vi "Set Offset.vi"(8 "error in (no error)":errorcluster, 11 "NeedleValve in":refnum<class "NeedleValve.lvclass">) -> (0 "error out":errorcluster, 3 "NeedleValve out":refnum<class "NeedleValve.lvclass">)   [LabVIEW 2019, in "NeedleValve.lvclass"]
uses:
  NeedleValve.lvclass
  NeedleValve.lvclass/NeedleValve.ctl
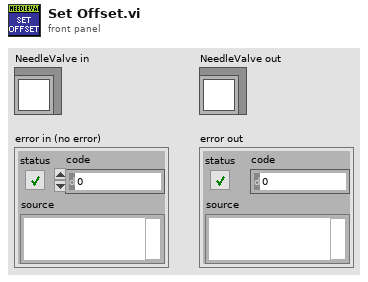
[diagram p1: front panel]
types:
  T1 = typedef "Needle Valve Data.ctl" = cluster{"Engine State":T2, "StateValveModbus":T3, "Alarms":T4, "RAW":i32, "Angele":dbl, "Step":i32, "Encoder":i32, "Kinematic":T5, "Limits":T6, "EncoderMax":i32, "Counter Max Dont Update":i32, "EncoderMin":i32, "Counter Min Dont Update":i32, "Prepere Counter":i32, "STEP INIT":i32, "offset - Angel":dbl}
  T2 = typedef "MB_ENGINE.lvclass/Engine State.ctl" = u16
  T3 = typedef "Needle Valve State.ctl" = enum16{"STOPED", "CLOSED", "OPENED", "OPENING", "CLOSING", "FULL_CLOSE", "PREP_OPEN"}
  T4 = typedef "MB_ENGINE.lvclass/Engine Alarms.ctl" = cluster{"OL":bool, "TF":bool, "STL":bool, "OCP":bool, "CPUV":bool, "UVLO":bool, "SPI_ERROR":bool, "Fault":bool, "OL 2":bool, "TF 2":bool, "STL 2":bool, "OCP 2":bool, "CPUV 2":bool, "UVLO 2":bool, "reserved":bool, "InitDone":bool}
  T5 = typedef "MB_ENGINE.lvclass/Settings.ctl" = cluster{"ACC Steps Per Sec^2":u16, "DEC Steps Per Sec^2":u16, "Min Velosity Step Per Sec":u16, "Max Velosity Step Per Sec":u16, "MicroStep":u16}
  T6 = typedef "MB_ENGINE.lvclass/Limits Status.ctl" = cluster{"Fault 2 Switch":bool, "Fault 1 Switch":bool, "Center(Home)":bool, "Lower Limit":bool, "Upper Limit":bool}
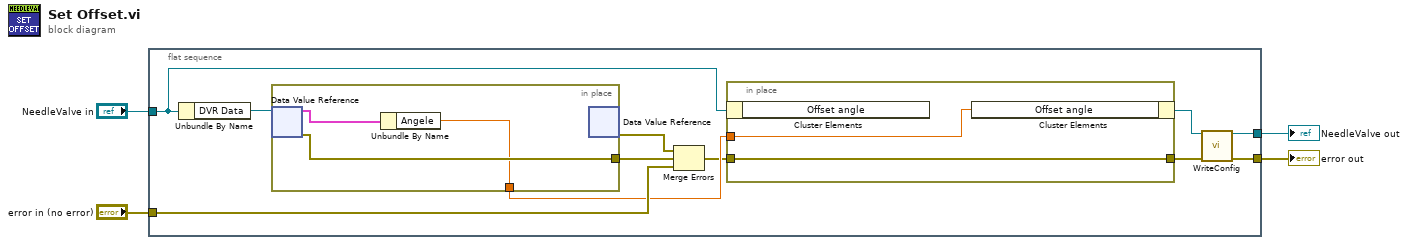
[diagram p0: block diagram]
diagram:
  n1 = flat-sequence {
    tunnel: "error in (no error)" -> [w15]
    tunnel: [w12] -> w2
    tunnel: [w11] -> w3
    tunnel: "NeedleValve in" -> [w9]
    frame #0 {
      n2 = Unbundle By Name(w9) -> ("DVR Data"=w8:refnum<data-value>)
      n3 = in-place {
        in-place-border: [w18] -> w6
        in-place-border: [w16] -> w10
        n4 = in-place-dvr #1(w8) -> (w17:T1, w18:errorcluster)
        n5 = Unbundle By Name(w17) -> ("Angele"=w16:dbl)
        n6 = in-place-dvr #1() -> (w5:errorcluster)  [unwired: 1 in, 1 out]
      }
      n7 = Merge Errors(w5, w6, w15) -> (w7:errorcluster)
      n8 = in-place {
        in-place-border: w7 -> [w20]
        in-place-border: [w20] -> w14
        in-place-border: w10 -> [w19]
        n9 = in-place-cluster #2(w9) -> ()  [unwired: 1 out]
        n10 = in-place-cluster #2("Offset angle"=w19) -> (w13:refnum<class "NeedleValve.lvclass">)
      }
      n11 = call-dynamic "WriteConfig.vi"("reference in"=w13, "error in (no error)"=w14) -> ("reference out"=w12:refnum<class "NeedleValve.lvclass">, "error out"=w11:errorcluster)  [unwired: 12 in]
    }
  }
  "error out" <- w3
  "NeedleValve out" <- w2
